vi "Read_Sonar.vi"(0 "error in":errorcluster, 3 "node":string) -> (1 "error out":errorcluster, 4 "Point Cloud":T1)   [LabVIEW 2010]
doc: "This VI returns point cloud from the head sonar readings"
panel:
  out "Reply":string
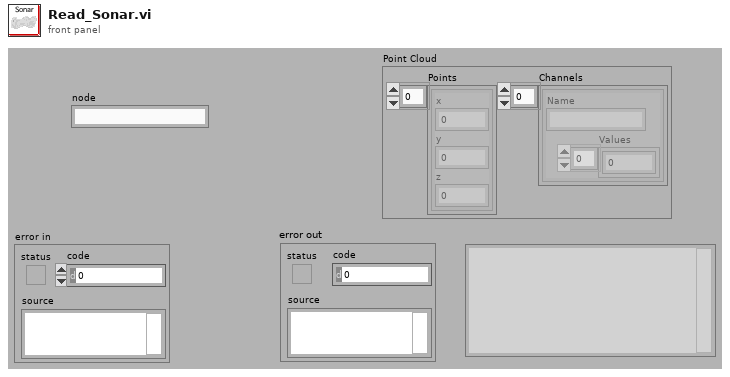
[diagram p1: front panel]
types:
  T1 = cluster{"Points":cluster{"x":sgl, "y":sgl, "z":sgl}[], "Channels":cluster{"Name":string, "Values":sgl[]}[]}
  T2 = typedef "_ROSControl.ctl" = cluster{"topic port":u16, "Node":string, "topic":string, "type":string, "node port":u32, "error ":errorcluster, "Direction":T3, "APIs":string[]}
  T3 = typedef "_ROSDirection.ctl" = enum16{"Node", "Publisher", "Subscriber", "Service Client"}
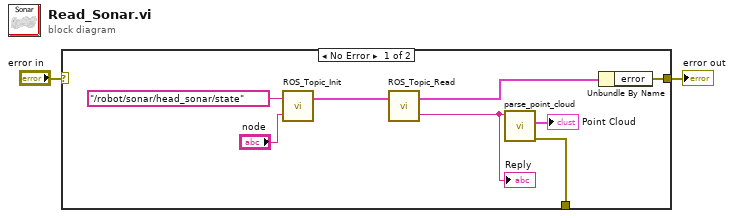
[diagram p0: block diagram]
diagram:
  n1 = case shown="No Error" "error in" {
    selector: "error in" -> [_ w11]
    tunnel: [w10 w11] -> w2
    tunnel: [w3 _] -> _
    frame No Error {
      n2 = call <userlib>:"ROS_Topic_Init.vi"("node"="node", "topic"="/robot/sonar/head_sonar/state") -> ("ROS out"=w7:T2)  [unwired: 1 in]
      n3 = call <userlib>:"ROS_Topic_Read.vi"("ROS in"=w7) -> ("Reply"=w5:string, "ROS out"=w6:T2)  [unwired: 1 in]
      "Reply" <- w5
      n4 = call <userlib>:"parse_point_cloud.vi"("msg in"=w5) -> ("error out"=w3:errorcluster, "Point Cloud"=→"Point Cloud":T1)  [unwired: 3 in, 2 out]
      n5 = Unbundle By Name(w6) -> ("error"=w10:errorcluster)
    }
    frame Error {
    }
  }
  "error out" <- w2
